vi "read_params.vi"(8 "error in (no error)":errorcluster, 11 "KernelRidge in":refnum<class "KernelRidge.lvclass">) -> (0 "error out":errorcluster, 2 "params":T1={"alpha"={"alpha_type"="float", "alpha_float"=1.0, "alpha_list"=[]}, "kernel"="linear", "gamma"={"gamma_type"="None", "gamma_float"=0.0}, "degree"=3.0, "coef0"=1.0}, 3 "KernelRidge out":refnum<class "KernelRidge.lvclass">)   [LabVIEW 2020, in "KernelRidge.lvclass"]
uses:
  KernelRidge.lvclass
  Controls/kernel_ridge_params.ctl
  KernelRidge.lvclass/KernelRidge.ctl
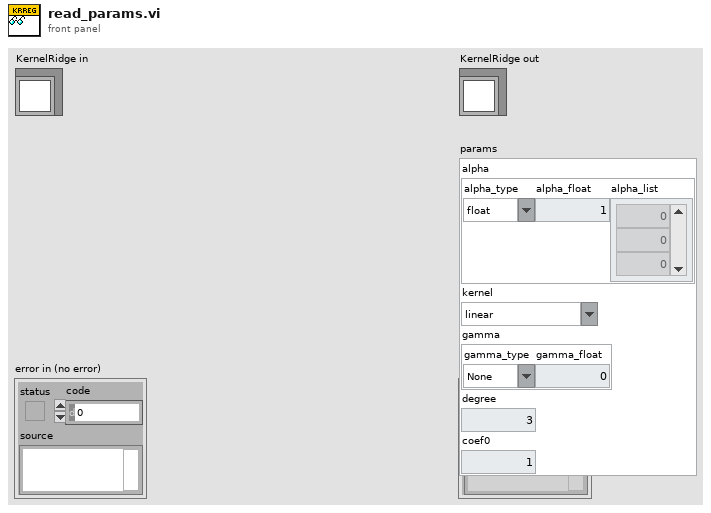
[diagram p1: front panel]
types:
  T1 = typedef "kernel_ridge_params.ctl" = cluster{"alpha":cluster{"alpha_type":string, "alpha_float":dbl, "alpha_list":dbl[]}, "kernel":string, "gamma":cluster{"gamma_type":string, "gamma_float":dbl}, "degree":dbl, "coef0":dbl}
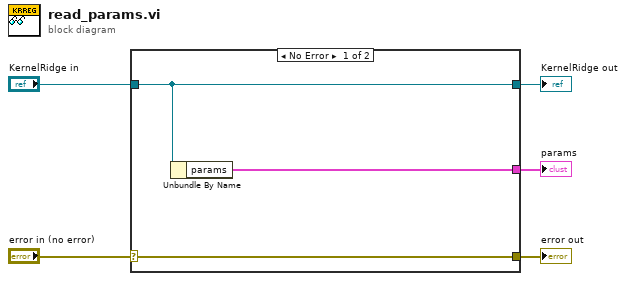
[diagram p0: block diagram]
diagram:
  n1 = case shown="No Error" "error in (no error)" {
    selector: "error in (no error)" -> [w8 w9]
    tunnel: [w8 w9] -> w4
    tunnel: [w7 w10] -> w2
    tunnel: "KernelRidge in" -> [w7 w10]
    tunnel: [w6 _] -> w1
    frame No Error {
      n2 = Unbundle By Name(w7) -> ("params"=w6:T1)
    }
    frame Error {
    }
  }
  "error out" <- w4
  "KernelRidge out" <- w2
  "params" <- w1
